vi "is_TMS_bit.vi"(2 "Mi (0 indexed)":i32) -> (7 "TMS bit":bool)   [LabVIEW 2015]
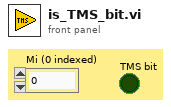
[diagram p1: front panel]
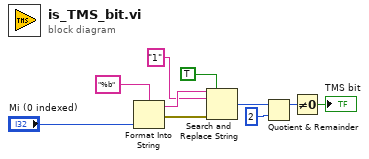
[diagram p0: block diagram]
diagram:
  n1 = Format Into String(format string="%b", "Mi (0 indexed)") -> (resulting string=w9:string, error out=w4:errorcluster)  [unwired: 2 in]
  n2 = Search and Replace String(replace all?=TRUE ("replace all? (F)"), input string=w9, search string="1", error in=w4) -> (number of replacements=w6:i32)  [unwired: 4 in, 3 out]
  n3 = Quotient & Remainder(x=w6, y=2) -> (x-y*floor(x/y)=w2:i32)  [unwired: 1 out]
  n4 = Not Equal To 0?(x=w2) -> (x != 0?=→"TMS bit":bool)
